vi "teleop_Moteur_Independant_vecteur.vi"(11 "SwerveDrive":T1) -> (3 "result":bool)   [LabVIEW 2018]
doc: "Les axes X and Y sont les deux axes qui font avancer le robot. X est horizontal et Y vertical selon le pilote.\nL'axez Z est l'axe qui permet au pilote de tourner en avançant dans une direction.\nLes boutons gauche et droite permettent au robot de tourner sur lui-même vers la gauche ou vers la droite selon quel bouton est actif.\n\nLe code vérifie que les roues sont dans le bon angle avant de faire avancer le robot."
uses:
  SwerveDrive.ctl
  MyGlobal.vi
  <vilib>/addons/control/pid/pid.llb/PID (DBL).vi
  <vilib>/addons/control/pid/NI_PID_pid.lvlib
panel:
  out "2":dbl
  out "3":dbl
  out "0":dbl
  out "1":dbl
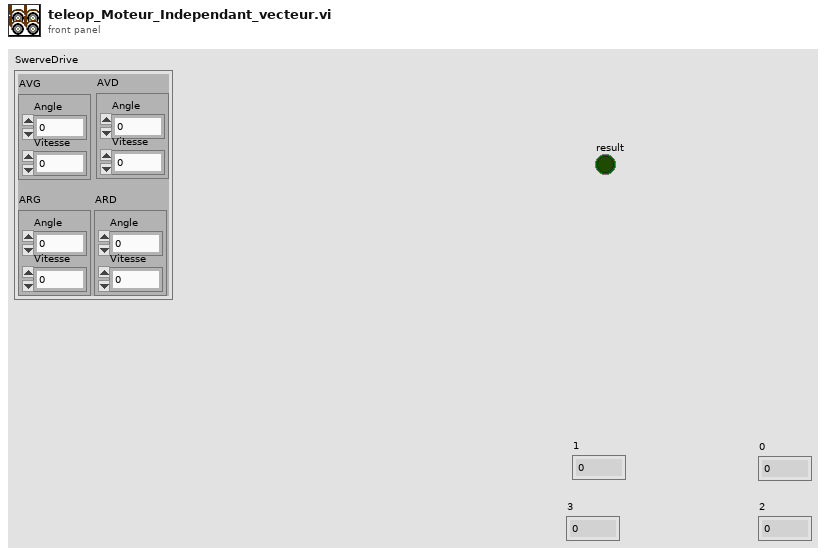
[diagram p1: front panel]
types:
  T1 = typedef "SwerveDrive.ctl" = cluster{"AVD":cluster{"Angle":dbl, "Vitesse":dbl}, "AVG":cluster{"Angle":dbl, "Vitesse":dbl}, "ARG":cluster{"Angle":dbl, "Vitesse":dbl}, "ARD":cluster{"Angle":dbl, "Vitesse":dbl}}
  T2 = cluster{"proportional gain (Kc)":dbl, "integral time (Ti, min)":dbl, "derivative time (Td, min)":dbl}
  T3 = typedef "Face Avant.ctl" = enum16{"0-1", "1-2", "2-3", "3-0"}
  T4 = typedef "WPI_EncoderDevRef.ctl" = cluster{"DevStatus":errorcluster, "EncoderIndex":T5, "CounterIndex":T6, "DistancePerCount":dbl, "Decoding Type":T7}
  T5 = typedef "FPGA_EncoderIdx.ctl" = enum8{"Enc 0", "Enc 1", "Enc 2", "Enc 3", "Enc 4", "Enc 5", "Enc 6", "Enc 7", "Invalid"}
  T6 = typedef "FPGA_CounterCtrSystemIndex.ctl" = enum8{"Ctr 0", "Ctr 1", "Ctr 2", "Ctr 3", "Ctr 4", "Ctr 5", "Ctr 6", "Ctr 7", "Invalid"}
  T7 = typedef "WPI_EncoderType.ctl" = enum16{"1x", "2x", "4x"}
  T8 = typedef "WPI_MotorControlDeviceRef.ctl" = cluster{"DeviceStatus":errorcluster, "Type":T9, "PWM":cluster{"PWM Channel":T10, "DeadBand":T11}, "CAN":cluster{"Device Number":u8, "SetOutput VI Ref":variant, "GetOutput VI Ref":variant, "Enable VI Ref":variant, "Disable VI Ref":variant, "Data":variant}, "Invert":bool, "DIO PWM":cluster{"PWM \"Enable\" Channel":T10, "DIOChannel":T12, "PWM Rate":dbl}}
  T9 = typedef "WPI_MotorControlType.ctl" = enum16{"PWM", "CAN", "DIO PWM"}
  T10 = typedef "FPGA_DIOPWMChannel.ctl" = enum8{"PWM 0", "PWM 1", "PWM 2", "PWM 3", "PWM 4", "PWM 5", "PWM 6", "PWM 7", "PWM 8", "PWM 9", "PWM MXP 0", "PWM MXP 1", "PWM MXP 2", "PWM MXP 3", "PWM MXP 4", "PWM MXP 5", "PWM MXP 6", "PWM MXP 7", "PWM MXP 8", "PWM MXP 9", "Invalid"}
  T11 = typedef "WPI_PWMDeadband.ctl" = cluster{"Name":string, "maxPositivePwm":i32, "minPositivePwm":i32, "centerPwm":i32, "maxNegativePwm":i32, "minNegativePwm":i32, "angularRange":u16}
  T12 = typedef "FPGA_DIOChannel.ctl" = enum8{"DIO 0", "DIO 1", "DIO 2", "DIO 3", "DIO 4", "DIO 5", "DIO 6", "DIO 7", "DIO 8", "DIO 9", "DIO MXP 0", "DIO MXP 1", "DIO MXP 2", "DIO MXP 3", "DIO MXP 4", "DIO MXP 5", "DIO MXP 6", "DIO MXP 7", "DIO MXP 8", "DIO MXP 9", "DIO MXP 10", "DIO MXP 11", "DIO MXP 12", "DIO MXP 13", "DIO MXP 14", "DIO MXP 15", "SPI Port CS1", "SPI Port CS2", "SPI Port CS3", "SPI Port MISO", "SPI Port MOSI", "Invalid"}
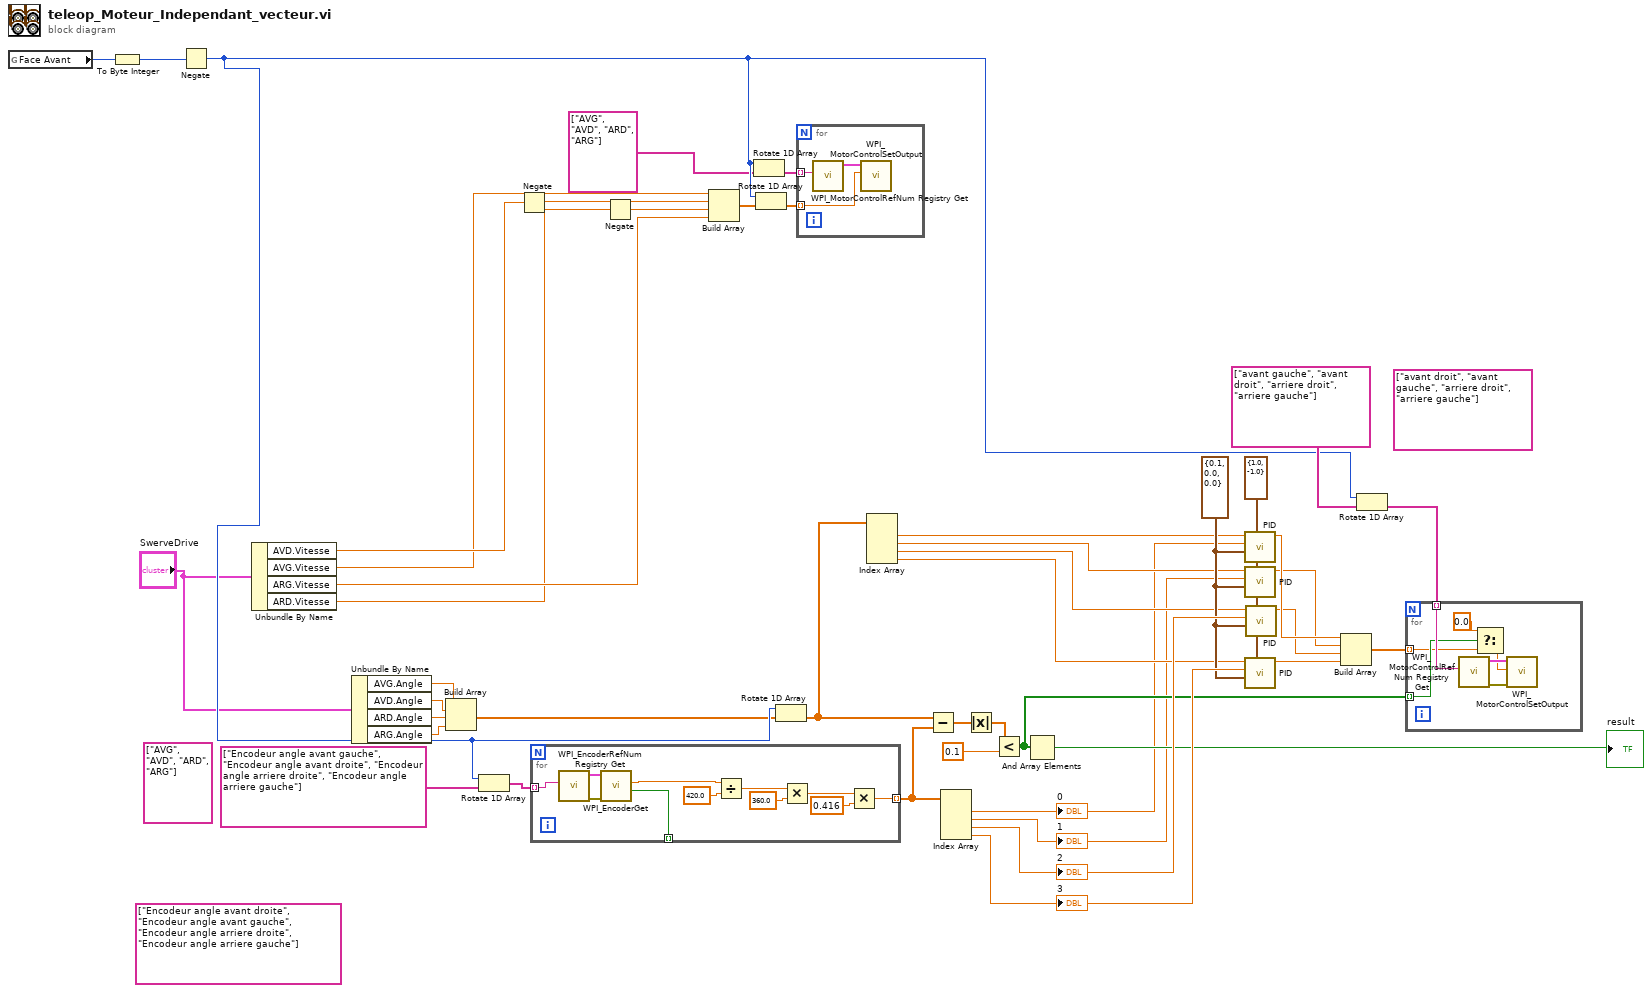
[diagram p0: block diagram]
diagram:
  (unwired) string[] ["avant droit", "avant gauche", "arriere droit", "arriere gauche"]
  (unwired) string[] ["AVG", "AVD", "ARD", "ARG"]
  (unwired) string[] ["Encodeur angle avant droite", "Encodeur angle avant gauche", "Encodeur angle arriere droite", "Encodeur angle arriere gauche"]
  w39 = cluster{"output high":dbl, "output low":dbl} {"output high"=1.0, "output low"=-1.0} ("output range")
  w38 = T2 {"proportional gain (Kc)"=0.1, "integral time (Ti, min)"=0.0, "derivative time (Td, min)"=0.0} ("PID gains")
  n1 = global read "MyGlobal.vi" "Face Avant"() -> (w25:T3)
  n2 = To Byte Integer(number=w25) -> (8bit integer=w24:i8)
  n3 = Negate(x=w24) -> (-x=w20:i8)
  n4 = Unbundle By Name("SwerveDrive") -> ("AVD.Vitesse"=w45:dbl, "AVG.Vitesse"=w44:dbl, "ARG.Vitesse"=w43:dbl, "ARD.Vitesse"=w42:dbl)
  n5 = Unbundle By Name("SwerveDrive") -> ("AVG.Angle"=w12:dbl, "AVD.Angle"=w11:dbl, "ARD.Angle"=w10:dbl, "ARG.Angle"=w9:dbl)
  n6 = Build Array(w12, w11, w10, w9) -> (w8:dbl[])
  n7 = Rotate 1D Array(1:string[] ["Encodeur angle avant gauche", "Encodeur angle avant droite", "Encodeur angle arriere droite", "Encodeur angle arriere gauche"], 2:w20) -> (0:w23:string[])
  n8 = Negate(x=w45) -> (-x=w17:dbl)
  n9 = for {
    tunnel: w23 -> [w47] mode=indexing
    tunnel: [w48] -> w37 mode=indexing
    tunnel: [w46] -> _ mode=indexing
    n10 = call <vilib>:"WPI_EncoderRefNum Registry Get.vi"("refnum name"=w47) -> ("error out"=w55:errorcluster, "EncoderDevRef"=w56:T4)  [unwired: 9 in]
    n11 = call <vilib>:"WPI_EncoderGet.vi"("error in (no error)"=w55, "EncoderDevRef"=w56) -> ("Direction"=w46:bool, "Distance"=w49:dbl)  [unwired: 4 in, 4 out]
    n12 = Divide(x=w49, y=420.0) -> (x/y=w50:dbl)
    n13 = Multiply(x=w50, y=360.0) -> (x*y=w54:dbl)
    n14 = Multiply(x=w54, y=0.416) -> (x*y=w48:dbl)
  }
  n15 = Negate(x=w42) -> (-x=w16:dbl)
  n16 = Build Array(w44, w17, w16, w43) -> (w18:dbl[])
  n17 = Rotate 1D Array(1:string[] ["AVG", "AVD", "ARD", "ARG"], 2:w20) -> (0:w15:string[])
  n18 = Rotate 1D Array(1:w18, 2:w20) -> (0:w14:dbl[])
  n19 = Rotate 1D Array(1:w8, 2:w20) -> (0:w7:dbl[])
  n20 = for {
    tunnel: w15 -> [w58] mode=indexing
    tunnel: w14 -> [w57] mode=indexing
    n21 = call <vilib>:"WPI_MotorControlRefNum Registry Get.vi"("refnum name"=w58) -> ("MotorControlDevRef"=w59:T8)  [unwired: 9 in, 1 out]
    n22 = call <vilib>:"WPI_MotorControlSetOutput.vi"("Output"=w57, "MotorControlDevRef"=w59) -> ()  [unwired: 7 in, 3 out]
  }
  n23 = Index Array(array=w7) -> (element #1=w6:dbl, element #2=w5:dbl, element #3=w4:dbl, element #4=w3:dbl)  [unwired: 4 in]
  n24 = Subtract(x=w7, y=w37) -> (x-y=w36:dbl[])
  n25 = Index Array(array=w37) -> (element #1=w2:dbl, element #2=w1:dbl, element #3=w41:dbl, element #4=w40:dbl)  [unwired: 4 in]
  "1" <- w1
  "0" <- w2
  "3" <- w40
  "2" <- w41
  n26 = Absolute Value(x=w36) -> (abs(x)=w35:dbl[])
  n27 = Less?(x=w35, y=0.1) -> (x < y?=w31:bool[])
  n28 = And Array Elements(Boolean array=w31) -> (logical AND=→"result":bool)
  n29 = call-poly <vilib>:"PID.vi"("output range"=w39, "PID gains"=w38, "process variable"=w2, "setpoint"=w6) -> ("output"=w29:dbl)  [unwired: 6 in, 1 out]
  n30 = call-poly <vilib>:"PID.vi"("output range"=w39, "PID gains"=w38, "process variable"=w1, "setpoint"=w5) -> ("output"=w27:dbl)  [unwired: 6 in, 1 out]
  n31 = call-poly <vilib>:"PID.vi"("output range"=w39, "PID gains"=w38, "process variable"=w40, "setpoint"=w3) -> ("output"=w26:dbl)  [unwired: 6 in, 1 out]
  n32 = call-poly <vilib>:"PID.vi"("output range"=w39, "PID gains"=w38, "process variable"=w41, "setpoint"=w4) -> ("output"=w28:dbl)  [unwired: 6 in, 1 out]
  n33 = Build Array(w29, w27, w28, w26) -> (w30:dbl[])
  n34 = Rotate 1D Array(1:string[] ["avant gauche", "avant droit", "arriere droit", "arriere gauche"], 2:w20) -> (0:w21:string[])
  n35 = for {
    tunnel: w21 -> [w64] mode=indexing
    tunnel: w31 -> [w61] mode=indexing
    tunnel: w30 -> [w60] mode=indexing
    n36 = call <vilib>:"WPI_MotorControlRefNum Registry Get.vi"("refnum name"=w64) -> ("error out"=w65:errorcluster, "MotorControlDevRef"=w66:T8)  [unwired: 9 in]
    n37 = Select(t=0.0 ("f"), s=w61, f=w60) -> (s? t:f=w62:dbl)
    n38 = call <vilib>:"WPI_MotorControlSetOutput.vi"("error in (no error)"=w65, "Output"=w62, "MotorControlDevRef"=w66) -> ()  [unwired: 6 in, 3 out]
  }
